vi "Remove All Nodes.vi"(8 "error in (no error)":errorcluster, 9 "Timeout(ms)":i64=10000, 11 "Simple Numeric Map Node Controller in":refnum<class "Simple Numeric Map Node Controller.lvclass">) -> (0 "error out":errorcluster, 3 "Simple Numeric Map Node Controller out":refnum<class "Simple Numeric Map Node Controller.lvclass">)   [LabVIEW 2024, in "Simple Numeric Map Node Controller.lvclass"]
uses:
  Simple Numeric Map Node Controller.lvclass
  Simple Numeric Map Node Controller.lvclass/Simple Numeric Map Node Controller.ctl
  011ac9d9-9998-4204-b831-e00158659893.vi
panel:
  out "Last State":T1(array[ring])
  out "None Stopped VI Refs":i32[](array[numeric])
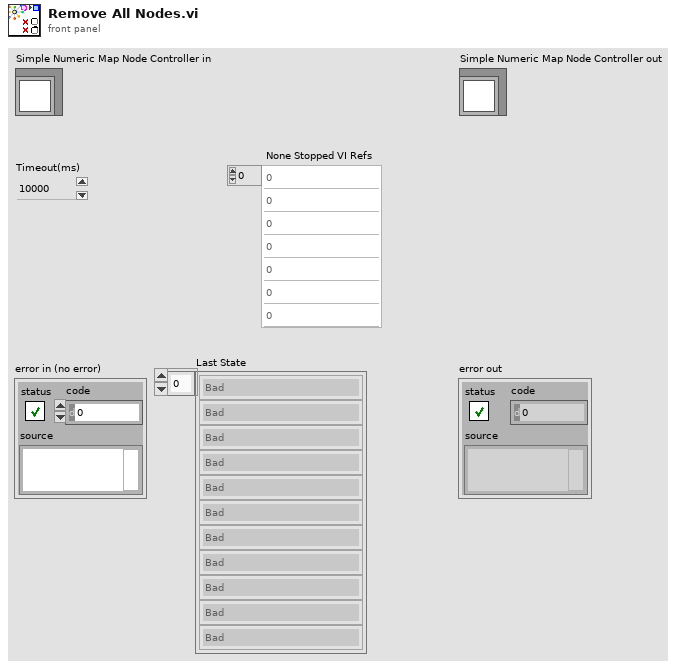
[diagram p1: front panel]
types:
  T1 = enum32{"Bad", "Idle", "Run top level", "Running"}[]
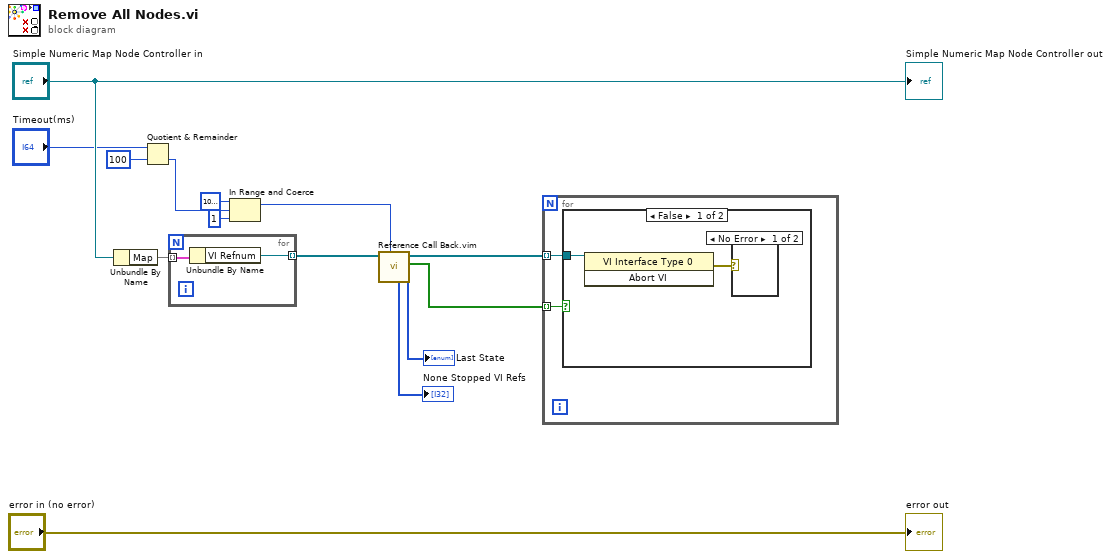
[diagram p0: block diagram]
diagram:
  n1 = Unbundle By Name("Simple Numeric Map Node Controller in") -> ("Map"=w9:map{i64, refnum<vi>})
  n2 = Quotient & Remainder(x="Timeout(ms)", y=i64 100) -> (floor(x/y)=w5:i64)  [unwired: 1 out]
  n3 = for {
    tunnel: w9 -> [w16] mode=indexing
    tunnel: [w15] -> w8 mode=indexing
    n4 = Unbundle By Name(w16) -> ("VI Refnum"=w15:refnum<vi>)
  }
  n5 = In Range and Coerce(upper limit=i64 1000000000, x=w5, lower limit=i64 1) -> (coerced(x)=w2:i64)  [unwired: 1 out]
  n6 = call "Reference Call Back.vim"("Waiting Loops"=w2, "VI Refnum In"=w8) -> ("Exec.State"=→"Last State":T1, "Terminated"=w12:bool[], "VI Refnum Out"=w11:refnum<vi>[], "None Stopped Refs"=→"None Stopped VI Refs":i32[])  [unwired: 6 in]
  n7 = for {
    tunnel: w11 -> [w17] mode=indexing
    tunnel: w12 -> [w18] mode=indexing
    n8 = case shown="False" w18 {
      tunnel: w17 -> [w20 _]
      frame False {
        n9 = invoke class="VI Interface Type 0" method="Abort VI"(reference=w20) -> (error out=w19:errorcluster)  [unwired: 2 in, 2 out]
        n10 = case shown="No Error" w19 {
          frame No Error {
          }
          frame Error {
          }
        }
      }
      frame True {
      }
    }
  }
  "error out" <- "error in (no error)"
  "Simple Numeric Map Node Controller out" <- "Simple Numeric Map Node Controller in"
